vi "Go To Field.vi"(8 "error in (no error)":errorcluster, 9 "Rate (Oe/s)":dbl=10.0, 10 "Target Field":dbl) -> (0 "error out":errorcluster)   [LabVIEW 2016]
uses:
  PPMS Global.vi
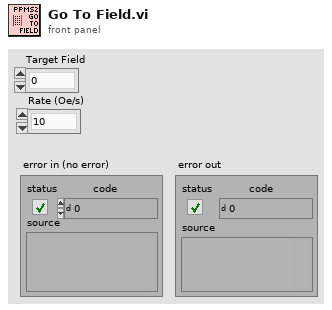
[diagram p1: front panel]
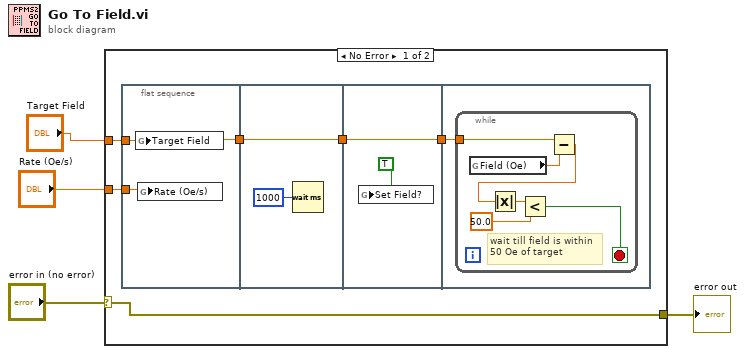
[diagram p0: block diagram]
diagram:
  n1 = case shown="No Error" "error in (no error)" {
    selector: "error in (no error)" -> [w10 w24]
    tunnel: [w10 w24] -> w3
    tunnel: "Rate (Oe/s)" -> [w9 _]
    tunnel: "Target Field" -> [w8 _]
    frame No Error {
      n2 = flat-sequence {
        tunnel: w9 -> [w12]
        tunnel: w8 -> [w11]
        tunnel: [w11] -> w7
        tunnel: w7 -> [w13]
        tunnel: [w13] -> w6
        tunnel: w6 -> [w15]
        tunnel: [w15] -> w5
        tunnel: w5 -> [w17]
        frame #0 {
          n3 = global write "PPMS Global.vi" "Target Field"(w11) -> ()
          n4 = global write "PPMS Global.vi" "Rate (Oe/s)"(w12) -> ()
        }
        frame #1 {
          n5 = Wait (ms)(milliseconds to wait=u32 1000) -> ()  [unwired: 1 out]
        }
        frame #2 {
          n6 = global write "PPMS Global.vi" "Set Field?"(TRUE ("Set Field?")) -> ()
        }
        frame #3 {
          n7 = while {
            tunnel: w17 -> [w22]
            stop <- w18 stop-if-true
            # "wait till field is within\n50 Oe of target"
            n8 = global read "PPMS Global.vi" "Field (Oe)"() -> (w23:dbl)
            n9 = Subtract(x=w22, y=w23) -> (x-y=w21:dbl)
            n10 = Absolute Value(x=w21) -> (abs(x)=w20:dbl)
            n11 = Less?(x=w20, y=50.0) -> (x < y?=w18:bool)
          }
        }
      }
    }
    frame Error {
    }
  }
  "error out" <- w3
